vi "Refine Corner.vi"(4 "ZeroZone [px]":i32=-1, 6 "WinSize [px]":i32=11, 8 "error in":errorcluster, 9 "pointY guess [px]":sgl=42.0, 10 "pointX guess [px]":sgl=52.0, 11 "Intensity Graph":refnum<vi>) -> (0 "error out":errorcluster, 1 "refined pointY":sgl, 2 "refiend pointX":sgl, 3 "success":i32)   [LabVIEW 2023, in "tg-analysis.lvlib"]
uses:
  gitlab/thermography-analysis/tg-analysis.lvlib
  build/x64/Release/MarkerLib-LabVIEW-Wrapper.dll
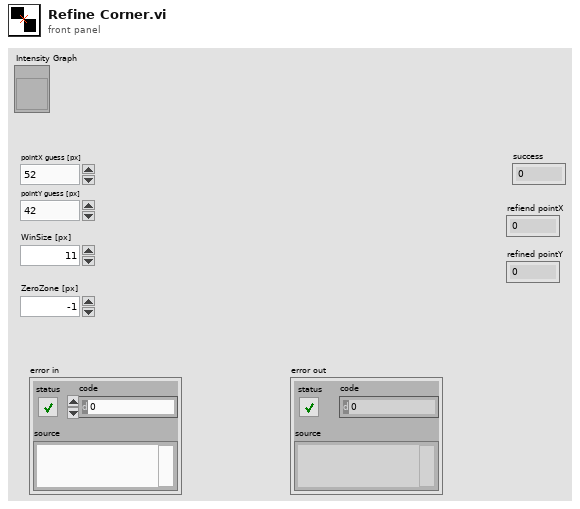
[diagram p1: front panel]
types:
  T1 = cluster{"Width":u16, "Style":enum32{"Solid", "Dash", "Dot", "DashDot", "DashDotDot"}}
  T2 = typedef "LVPoint32TypeDef.ctl" = cluster{"Horizontal":i32, "Vertical":i32}
  T3 = typedef "LVRectTypeDef.ctl" = cluster{"Left":i16, "Top":i16, "Right":i16, "Bottom":i16}
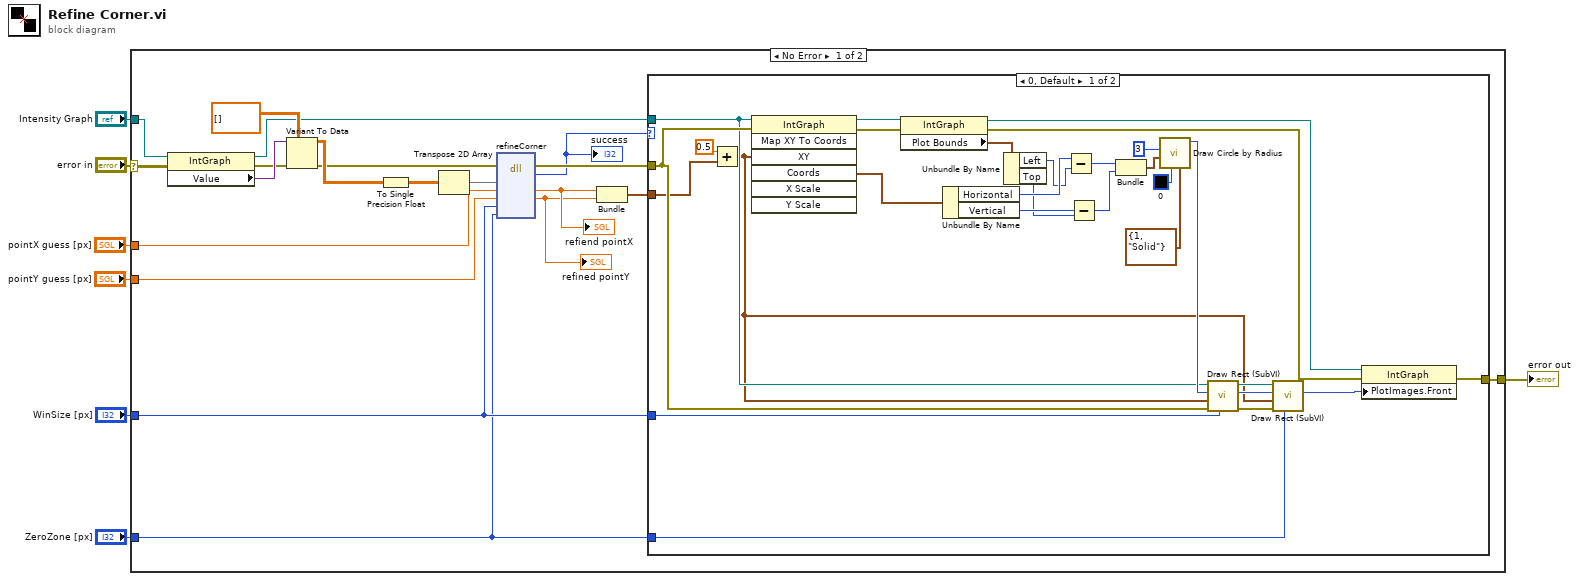
[diagram p0: block diagram]
diagram:
  n1 = case shown="No Error" "error in" {
    selector: "error in" -> [w18 w58]
    tunnel: [w14 w58] -> w7
    tunnel: "pointX guess [px]" -> [w26 _]
    tunnel: "pointY guess [px]" -> [w25 _]
    tunnel: "WinSize [px]" -> [w23 _]
    tunnel: "ZeroZone [px]" -> [w22 _]
    tunnel: "Intensity Graph" -> [w20 _]
    frame No Error {
      n2 = property class="IntGraph"(reference=w20, error in=w18) -> (reference out=w8:refnum<vi>, error out=w12:errorcluster, "Value"=w13:variant)
      n3 = Variant To Data(error in=w12, type=dbl[][] [], Variant=w13) -> (data=w10:dbl[][], error out=w9:errorcluster)
      n4 = To Single Precision Float(number=w10) -> (single precision float=w21:sgl[][])
      n5 = Transpose 2D Array(2D array=w21) -> (transposed array=w19:sgl[][])
      n6 = dll-call lib="D:/git/MarkerLib-LabVIEW-Wrapper/build/x64/Release/MarkerLib-LabVIEW-Wrapper.dll" fn="refineCorner"(error in=w9, "image"=w19, "pointX"=w26, "pointY"=w25, "winSize"=w23, "zeroZone"=w22) -> (error out=w27:errorcluster, "success"=w24:i32, "pointX"=w17:sgl, "pointY"=w16:sgl)  [unwired: 5 in, 1 out]
      "success" <- w24
      "refined pointY" <- w16
      "refiend pointX" <- w17
      n7 = Bundle("pointX"=w17, "pointY"=w16) -> (w15:cluster{"pointX":sgl, "pointY":sgl})  [unwired: 1 in]
      n8 = case shown="0, Default" w24 {
        tunnel: w27 -> [w39 w57]
        tunnel: w23 -> [w37 _]
        tunnel: w22 -> [w33 _]
        tunnel: w15 -> [w30 _]
        tunnel: [w32 w57] -> w14
        tunnel: w8 -> [w31 _]
        frame 0, Default {
          n9 = Add(x=sgl 0.5 ("pointX"), y=w30) -> (x+y=w28:cluster{"pointX":sgl, "pointY":sgl})
          n10 = invoke on="Invoke Node" class="IntGraph" method="Map XY To Coords"(reference=w31, error in=w39, "XY"=w28) -> (reference out=w53:refnum<vi>, error out=w52:errorcluster, "Coords"=w50:T2)  [unwired: 4 in, 4 out]
          n11 = property class="IntGraph"(reference=w53, error in=w52) -> (reference out=w41:refnum<vi>, error out=w40:errorcluster, "Plot Bounds"=w51:T3)
          n12 = Unbundle By Name(w50) -> ("Horizontal"=w49:i32, "Vertical"=w47:i32)
          n13 = Unbundle By Name(w51) -> ("Left"=w48:i16, "Top"=w46:i16)
          n14 = Subtract(x=w49, y=w48) -> (x-y=w44:i32)
          n15 = Subtract(x=w47, y=w46) -> (x-y=w43:i32)
          n16 = Bundle(w44, w43) -> (w45:cluster{i32, i32})  [unwired: 1 in]
          n17 = call <vilib>:"Draw Circle by Radius.vi"("pen"=T1 {"Width"=1, "Style"=enum."Solid"}, "color(black)"=u32 0, "pixel center"=w45, "radius"=i16 3) -> ("new picture"=w42:picture)  [unwired: 7 in]
          n18 = call "Draw Rect (SubVI).vi"("WinSize [px]"=w37, "error in (no error)"=w39, "Cluster"=w28, "new picture in"=w42, "IntensityGraph in"=w31) -> ("error out"=w38:errorcluster, "new picture out"=w35:picture, "IntensityGraph out"=w36:refnum<vi>)  [unwired: 4 in]
          n19 = call "Draw Rect (SubVI).vi"("WinSize [px]"=w33, "error in (no error)"=w38, "Cluster"=w28, "new picture in"=w35, "IntensityGraph in"=w36) -> ("new picture out"=w34:picture)  [unwired: 4 in, 2 out]
          n20 = property on="Property Node" class="IntGraph"(reference=w41, error in=w40, "PlotImages.Front"=w34) -> (error out=w32:errorcluster)  [unwired: 1 out]
        }
        frame 1 {
        }
      }
    }
    frame Error {
    }
  }
  "error out" <- w7
